vi "Write RRT Parameters.vi"(8 "error in (no error)":errorcluster, 10 "RRT Parameters":T1={"threshold"=120.0, "Step"=120.0, "GoalProb"=0.1, "WayPointProb"=0.6} {"WayPointProb" format="%#_13g"; "GoalProb" format="%#_13g"}, 11 "Parameters in":refnum<class "Parameters.lvclass">) -> (0 "error out":errorcluster, 3 "Parameters out":refnum<class "Parameters.lvclass">)   [LabVIEW 2023, in "Parameters.lvclass"]
uses:
  Parameters.lvclass
  Game_class/PathPlanning/Path Planning/RRT/RRTParameters.ctl
  Parameters.lvclass/Parameters.ctl
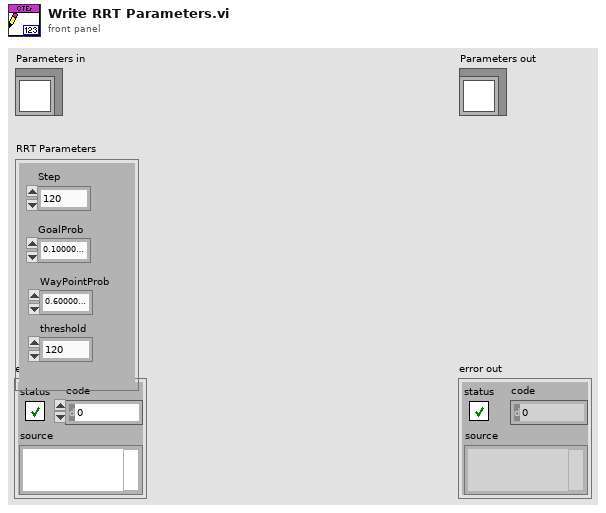
[diagram p1: front panel]
types:
  T1 = typedef "RRTParameters.ctl" = cluster{"threshold":sgl, "Step":sgl, "GoalProb":sgl, "WayPointProb":sgl}
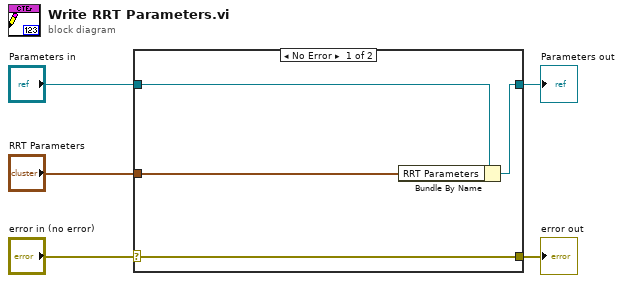
[diagram p0: block diagram]
diagram:
  n1 = case shown="No Error" "error in (no error)" {
    selector: "error in (no error)" -> [w9 w10]
    tunnel: [w9 w10] -> w4
    tunnel: [w7 w11] -> w2
    tunnel: "Parameters in" -> [w8 w11]
    tunnel: "RRT Parameters" -> [w6 _]
    frame No Error {
      n2 = Bundle By Name(cluster=w8, "RRT Parameters"=w6) -> (w7:refnum<class "Parameters.lvclass">)
    }
    frame Error {
    }
  }
  "error out" <- w4
  "Parameters out" <- w2
